vi "test Reading Slot Configuration.vi"(8 "error in (no error)":errorcluster, 11 "TestCase in":refnum<class "Scan Engine Unit Tests.lvclass">=refnum) -> (0 "error out":errorcluster, 3 "TestCase out":refnum<class "Scan Engine Unit Tests.lvclass">)   [LabVIEW 2026, in "Scan Engine Unit Tests.lvclass"]
uses:
  Scan Engine Unit Tests.lvclass
  <vilib>/NI VeriStand/Custom Device Tools/Custom Device Utility Library/Custom Device Utility Library.lvlib
  Shared/Globals/Scan Engine GUIDs.vi
  Shared/SEECD Shared.lvlib
  System Explorer/SEECD System Explorer.lvlib
  System Explorer/Type Defs/Slot Programming Mode.ctl
  NationalInstruments.VeriStand.SystemDefinitionAPI
  <vilib>/NI VeriStand/Custom Device Tools/Custom Device Utility Library/NI VeriStand - Search for Item by GUID.vi
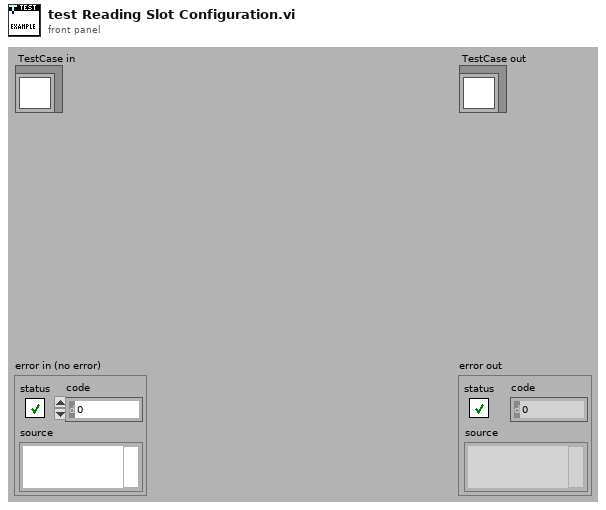
[diagram p1: front panel]
types:
  T1 = typedef "SEECD System Explorer.lvlib/Slot Programming Mode.ctl" = enum16{"Don't Modify", "Scan Engine", "LabVIEW FPGA", "NI-DAQmx"}
  T2 = typedef "Custom Device API.lvlib/Custom Device Item Ref.ctl" = u64
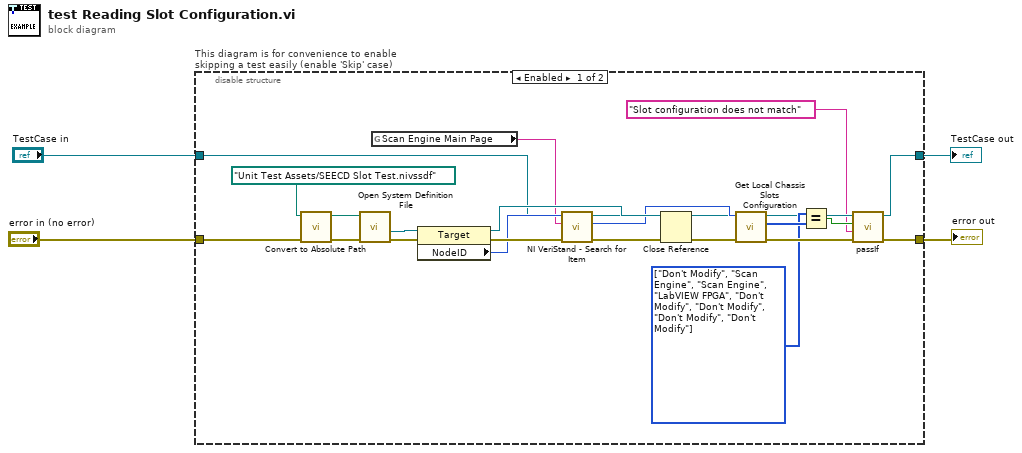
[diagram p0: block diagram]
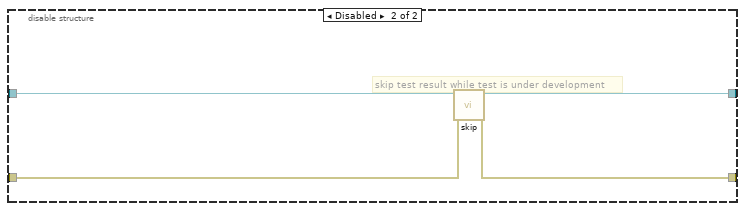
[diagram p2: hidden frame]
diagram:
  n1 = disable-structure "This diagram is for convenience to enable skipping a test easily (enable 'Skip' case)" shown="Enabled" {
    disable-tunnel: "TestCase in" -> [w8 w29]
    disable-tunnel: [w7 w27] -> w1
    disable-tunnel: [w6 w28] -> w3
    disable-tunnel: "error in (no error)" -> [w25 w26]
    frame Enabled {
      w10 = T1[] [enum."Don't Modify", enum."Scan Engine", enum."Scan Engine", enum."LabVIEW FPGA", enum."Don't Modify", enum."Don't Modify", enum."Don't Modify", enum."Don't Modify"] items=["Don't Modify", "Scan Engine", "LabVIEW FPGA", "NI-DAQmx"] ("Slots Configuration")
      n2 = call "Convert to Absolute Path.vi"("error in"=w25, "path"=path "Unit Test Assets/SEECD Slot Test.nivssdf") -> ("error out"=w24:errorcluster, "absolute path"=w22:path)  [unwired: 8 in]
      n3 = call "Open System Definition File.vi"("error in"=w24, "path"=w22) -> ("error out"=w20:errorcluster, "target ref"=w21:refnum<k24>)  [unwired: 6 in, 2 out]
      n4 = global read "Scan Engine GUIDs.vi" "Scan Engine Main Page"() -> (w15:string)
      n5 = property class="Target"(reference=w21, error in=w20) -> (reference out=w16:refnum<k24>, error out=w19:errorcluster, "NodeID"=w18:u64)
      n6 = call-poly <vilib>:"NI VeriStand - Search for Item.vi"("error in"=w19, "Item GUID"=w15, "Section Ref in"=w18) -> ("error out"=w17:errorcluster, "Item Ref"=w13:T2)  [unwired: 5 in, 2 out]
      n7 = Close Reference(reference=w16, error in (no error)=w17) -> (error out=w14:errorcluster)
      n8 = call "Get Local Chassis Slots Configuration.vi"("error in (no error)"=w14, "Item Ref in"=w13) -> ("error out"=w12:errorcluster, "Slots Configuration"=w11:T1[])  [unwired: 7 in, 1 out]
      n9 = Equal?(x=w10, y=w11) -> (x = y?=w9:bool)
      n10 = call-dynamic "passIf.vi"("error in (no error)"=w12, "message (\"\")"="Slot configuration does not match" ("message (\"\")"), "pass"=w9, "TestCase in"=w8) -> ("error out"=w6:errorcluster, "TestCase out"=w7:refnum<class "Scan Engine Unit Tests.lvclass">)  [unwired: 6 in]
    }
    frame Disabled {
      # "skip test result while test is under development"
      n11 = call <vilib>:"skip.vi"("error in (no error)"=w26, "TestCase in"=w29) -> ("error out"=w28:errorcluster, "TestCase out"=w27:refnum<class "Scan Engine Unit Tests.lvclass">)  [unwired: 8 in]
    }
  }
  "error out" <- w3
  "TestCase out" <- w1
